vi "osciloscope.vi"() -> ()   [LabVIEW 2023]
doc: "Simulate a osciloscope VI"
uses:
  <vilib>/Utility/error.llb/DialogType.ctl
  <vilib>/Analysis/Matrix/Numeric/Conversions/Array To Matrix - RA.vi
  <vilib>/Analysis/Matrix/NI_Matrix.lvlib
panel:
  out "error out":errorcluster
  in  "error in (no error)":errorcluster
  in  "Stop":bool
  in  "Channel 2":bool
  in  "Y Position Channel-2":dbl(knob) scale=-5.0..5.0
  in  "X position":dbl(knob) step=1.0 scale=0.0..10.0
  in  "Mode":T1(ring)
  in  "Channel 1":bool
  in  "Y Position Channel-1":dbl(knob) scale=-5.0..5.0
  in  "Power":bool
  in  "Fetch":bool
  out "Scope":dbl[][](graph)
  # "Measurement"
  # "ON"
  # "OFF"
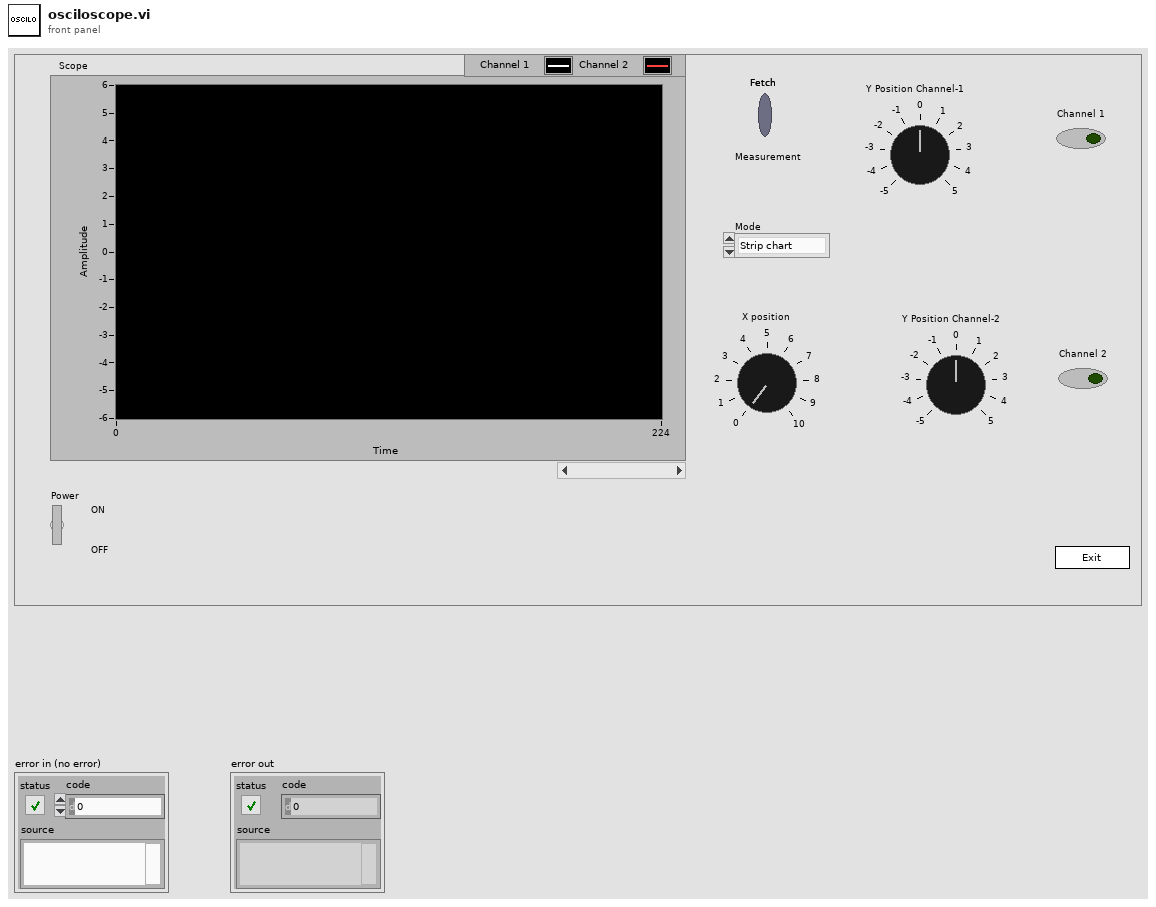
[diagram p1: front panel]
types:
  T1 = enum8{"Strip chart", "Scope chart", "Sweep chart"}
  T2 = cluster{"Power":bool, "Fetch":bool, "Channel 1":bool, "Channel 2":bool, "Y Channel 1":dbl, "Y Channel 2":dbl, "X Position":dbl, "x_value":i32}
  T3 = typedef "NI_Matrix.lvlib/RealMatrix.ctl" = dbl[][]
  T4 = typedef "DialogType.ctl" = u16
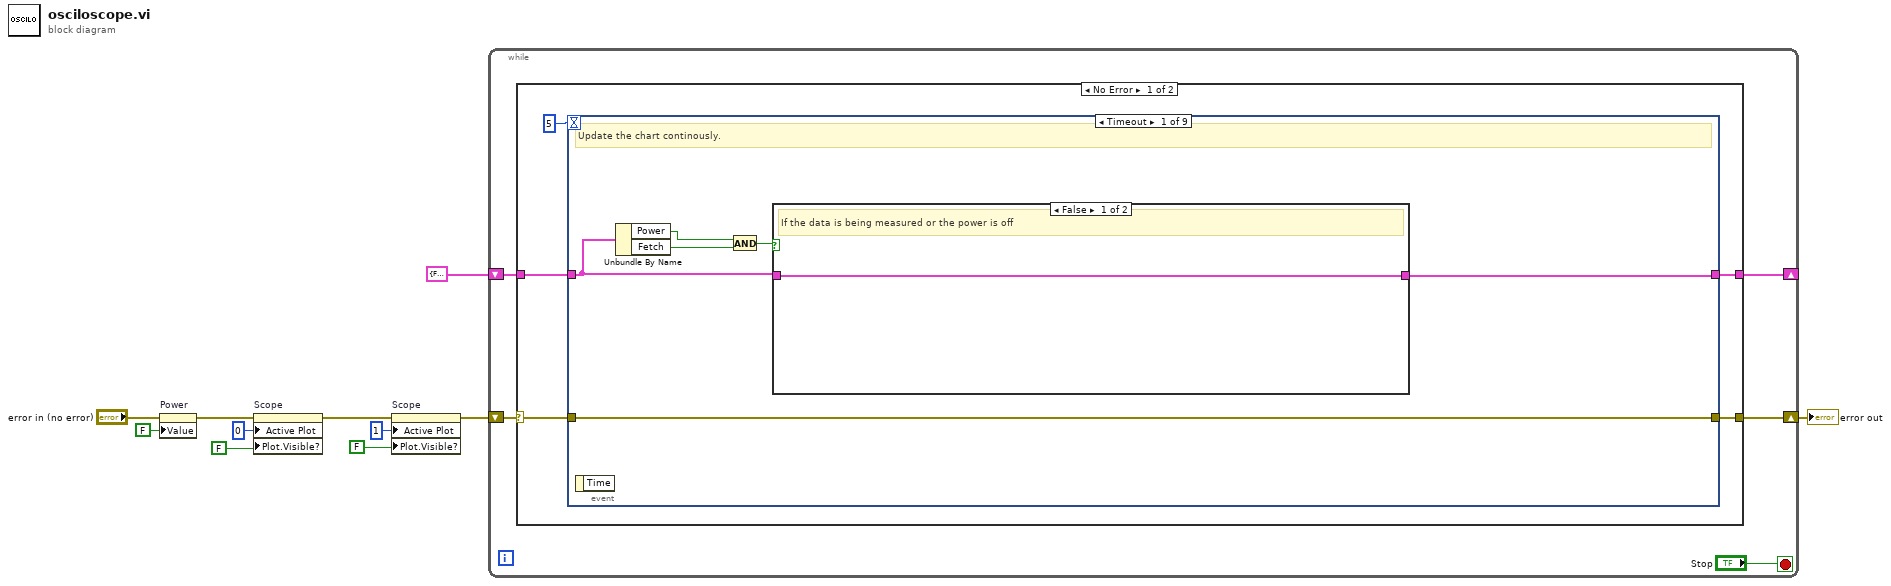
[diagram p0: block diagram]
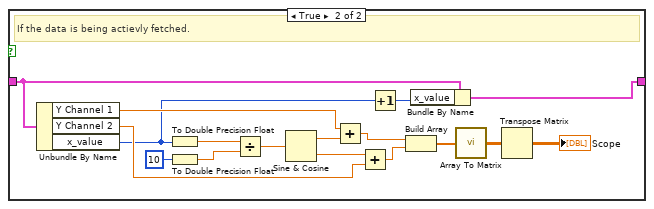
[diagram p2: hidden frame]
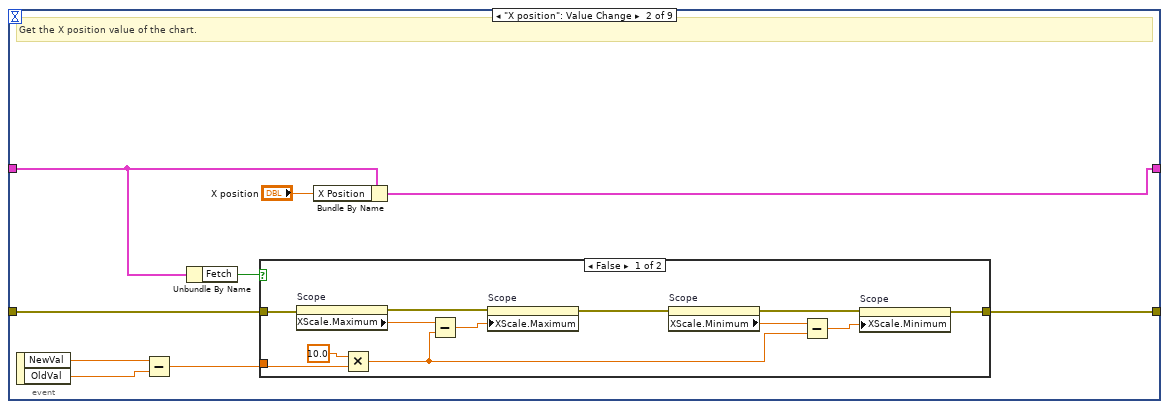
[diagram p3: hidden frame]
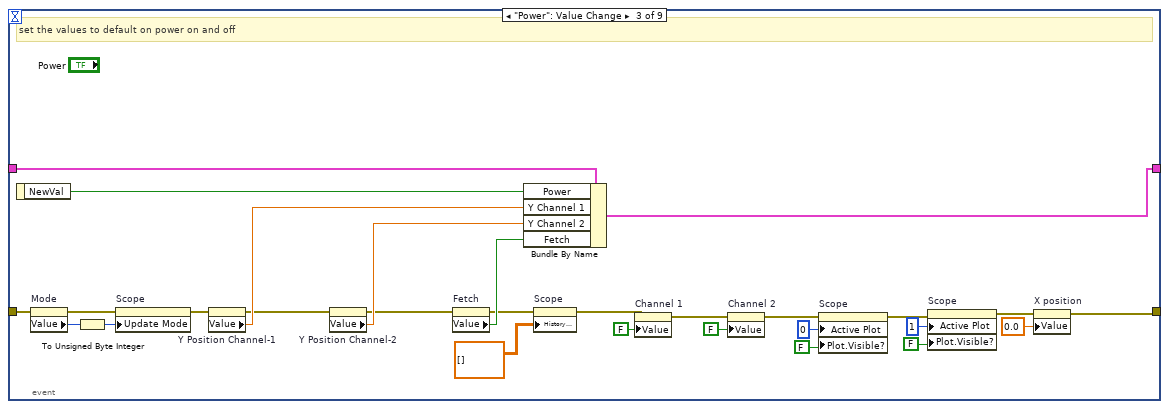
[diagram p5: hidden frame]
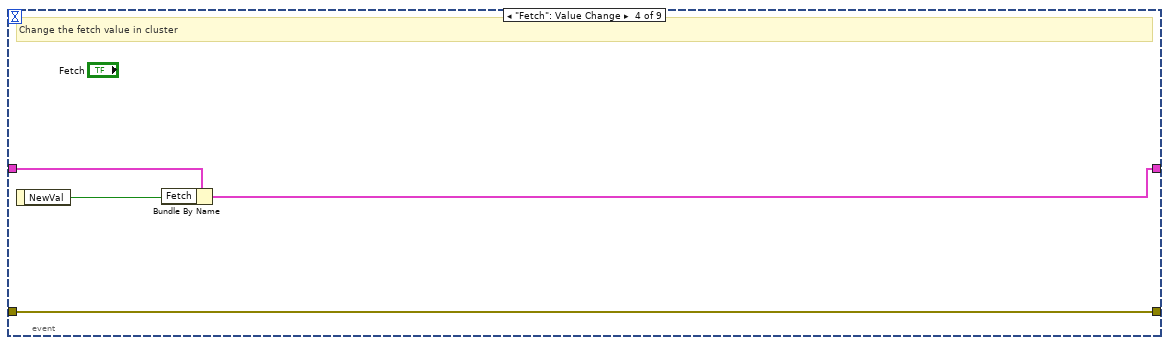
[diagram p6: hidden frame]
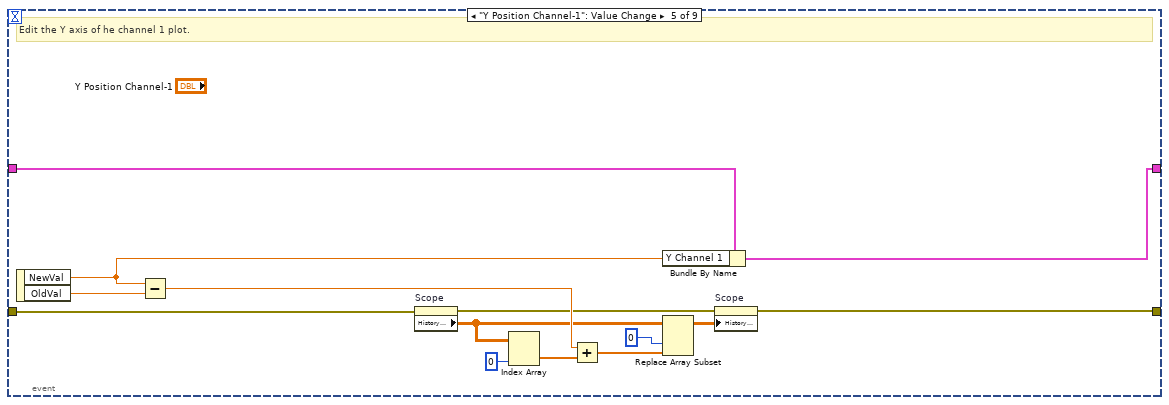
[diagram p7: hidden frame]
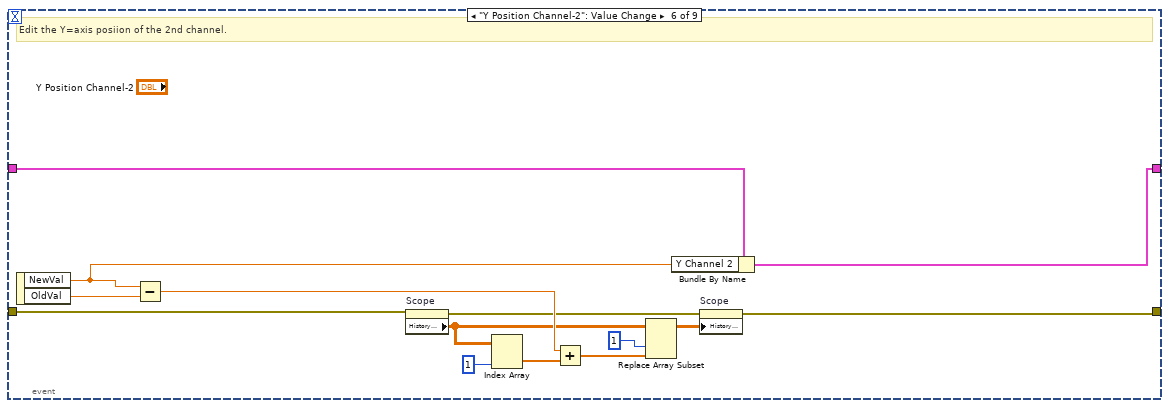
[diagram p8: hidden frame]
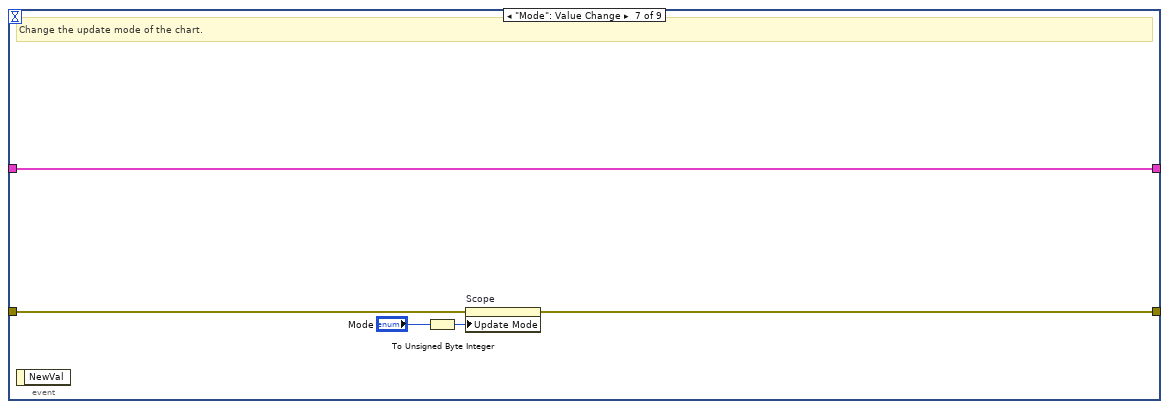
[diagram p9: hidden frame]
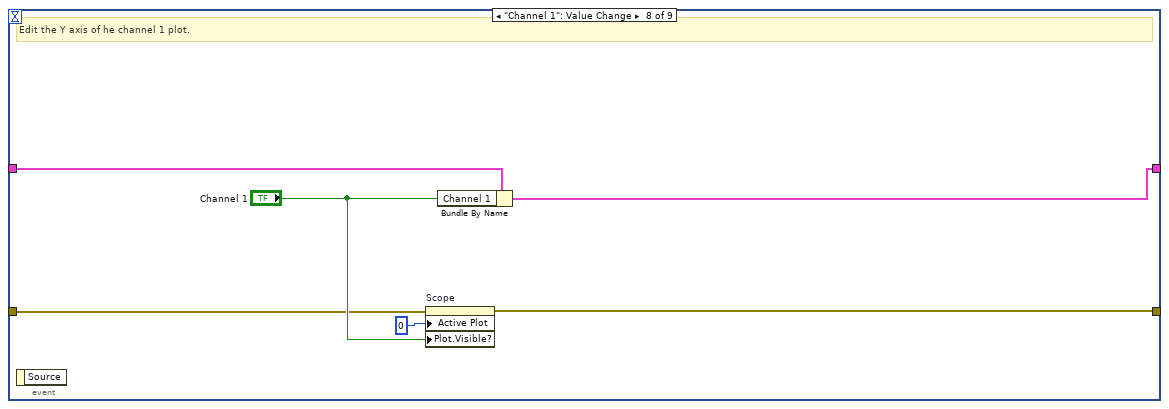
[diagram p10: hidden frame]
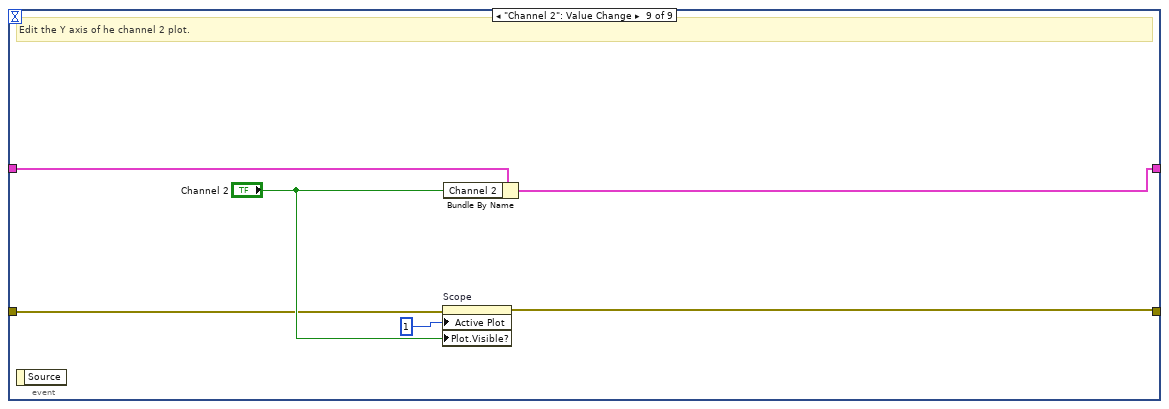
[diagram p11: hidden frame]
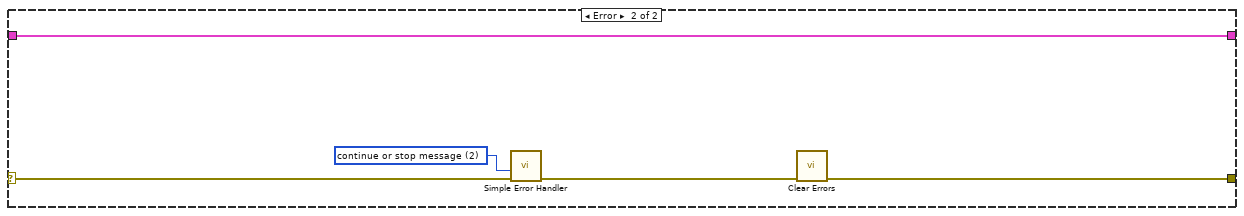
[diagram p12: hidden frame]
diagram:
  n1 = property on="Power" class="Bool (strict)"(error in="error in (no error)", "Value"=FALSE ("Power")) -> (error out=w4:errorcluster)  [unwired: 1 in, 1 out]
  n2 = property on="Scope" class="WFChart (strict)"(error in=w4, "Active Plot"=u32 0, "Plot.Visible?"=FALSE ("Plot.Visible")) -> (error out=w6:errorcluster)  [unwired: 1 in, 1 out]
  n3 = property on="Scope" class="WFChart (strict)"(error in=w6, "Active Plot"=u32 1, "Plot.Visible?"=FALSE ("Plot.Visible")) -> (error out=w3:errorcluster)  [unwired: 1 in, 1 out]
  n4 = while {
    shift-right: [w15] -> _
    shift-left: T2 {"Power"=FALSE, "Fetch"=TRUE, "Channel 1"=FALSE, "Channel 2"=FALSE, "Y Channel 1"=0.0, "Y Channel 2"=0.0, "X Position"=0.0, "x_value"=0} -> [w16]
    shift-right: [w12] -> w1
    shift-left: w3 -> [w13]
    stop <- "Stop" stop-if-true
    n5 = case shown="No Error" w13 {
      selector: w13 -> [w18 w148]
      tunnel: w16 -> [w20 w149]
      tunnel: [w19 w149] -> w15
      tunnel: [w17 w146] -> w12
      frame No Error {
        n6 = event shown="[0] Timeout" {
          selector: _ -> [_ _ _ _ _ _ _ _ _]
          dyn-events: _ -> [_ _ _ _ _ _ _ _ _]
          timeout: 5 ("milliseconds to wait") -> [_ _ _ _ _ _ _ _ _]
          tunnel: w20 -> [w27 w47 w95 w99 w110 w124 w131 w138 w144]
          tunnel: [w26 w54 w94 w98 w113 w127 w131 w137 w143] -> w19
          tunnel: w18 -> [w25 w50 w69 w96 w101 w115 w129 w134 w140]
          tunnel: [w25 w48 w68 w96 w100 w114 w128 w133 w139] -> w17
          event Timeout {
            # "Update the chart continously."
            n7 = event-data() -> ()  [unwired: 1 in, 1 out]
            n8 = Unbundle By Name(w27) -> ("Power"=w23:bool, "Fetch"=w22:bool)
            n9 = And(x=w23, y=w22) -> (x .and. y?=w24:bool)
            n10 = case shown="False" w24 {
              tunnel: w27 -> [w28 w32]
              tunnel: [w28 w31] -> w26
              frame False {
                # "If the data is being measured or the power is off"
              }
              frame True {
                # "If the data is being actievly fetched."
                n11 = Unbundle By Name(w32) -> ("Y Channel 1"=w34:dbl, "Y Channel 2"=w33:dbl, "x_value"=w29:i32)
                n12 = To Double Precision Float(number=w29) -> (double precision float=w43:dbl)
                n13 = To Double Precision Float(number=10 ("y")) -> (double precision float=w42:dbl)
                n14 = Divide(x=w43, y=w42) -> (x/y=w45:dbl)
                n15 = Sine & Cosine(0:w45) -> (1:w36:dbl, 2:w41:dbl)
                n16 = Add(x=w34, y=w36) -> (x+y=w37:dbl)
                n17 = Add(x=w41, y=w33) -> (x+y=w35:dbl)
                n18 = Increment(x=w29) -> (x+1=w30:i32)
                n19 = Build Array(w37, w35) -> (w39:dbl[])
                n20 = Bundle By Name(cluster=w32, "x_value"=w30) -> (w31:T2)
                n21 = call-poly <vilib>:"Array To Matrix.vi"("Real 1D Array"=w39) -> ("Real Matrix (Column Vector)"=w40:T3)
                n22 = Transpose Matrix(1:w40) -> (0:→"Scope":T3)
              }
            }
          }
          event "X position": Value Change {
            # "Get the X position value of the chart."
            n23 = event-data() -> ("NewVal"=w52:dbl, "OldVal"=w51:dbl)  [unwired: 1 in]
            n24 = Subtract(x=w52, y=w51) -> (x-y=w49:dbl)
            n25 = Unbundle By Name(w47) -> ("Fetch"=w46:bool)
            n26 = case shown="False" w46 {
              tunnel: w50 -> [w64 w67]
              tunnel: w49 -> [w62 _]
              tunnel: [w56 w67] -> w48
              frame False {
                n27 = property on="Scope" class="WFChart (strict)"(error in=w64) -> (error out=w63:errorcluster, "XScale.Maximum"=w65:dbl)  [unwired: 1 in, 1 out]
                n28 = Multiply(x=10.0, y=w62) -> (x*y=w55:dbl)
                n29 = Subtract(x=w65, y=w55) -> (x-y=w66:dbl)
                n30 = property on="Scope" class="WFChart (strict)"(error in=w63, "XScale.Maximum"=w66) -> (error out=w57:errorcluster)  [unwired: 1 in, 1 out]
                n31 = property on="Scope" class="WFChart (strict)"(error in=w57) -> (error out=w60:errorcluster, "XScale.Minimum"=w59:dbl)  [unwired: 1 in, 1 out]
                n32 = Subtract(x=w59, y=w55) -> (x-y=w58:dbl)
                n33 = property on="Scope" class="WFChart (strict)"(error in=w60, "XScale.Minimum"=w58) -> (error out=w56:errorcluster)  [unwired: 1 in, 1 out]
              }
              frame True {
              }
            }
            n34 = Bundle By Name(cluster=w47, "X Position"="X position") -> (w54:T2)
          }
          event "Power": Value Change {
            w70 = 0.0 items=["0", "1", "2", "3", "4", "5", "6", "7", "8", "9", "10"] ("X position")
            # "set the values to default on power on and off"
            n35 = event-data() -> ("NewVal"=w93:bool)  [unwired: 1 in]
            n36 = property on="Mode" class="Enum (strict)"(error in=w69) -> (error out=w88:errorcluster, "Value"=w89:T1)  [unwired: 1 in, 1 out]
            n37 = To Unsigned Byte Integer(number=w89) -> (unsigned 8bit integer=w90:u8)
            n38 = property on="Scope" class="WFChart (strict)"(error in=w88, "Update Mode"=w90) -> (error out=w83:errorcluster)  [unwired: 1 in, 1 out]
            n39 = property on="Y Position Channel-1" class="Knob (strict)"(error in=w83) -> (error out=w85:errorcluster, "Value"=w92:dbl)  [unwired: 1 in, 1 out]
            n40 = property on="Y Position Channel-2" class="Knob (strict)"(error in=w85) -> (error out=w86:errorcluster, "Value"=w91:dbl)  [unwired: 1 in, 1 out]
            n41 = property on="Fetch" class="Bool (strict)"(error in=w86) -> (error out=w84:errorcluster, "Value"=w87:bool)  [unwired: 1 in, 1 out]
            n42 = Bundle By Name(cluster=w95, "Power"=w93, "Y Channel 1"=w92, "Y Channel 2"=w91, "Fetch"=w87) -> (w94:T2)
            n43 = property on="Scope" class="WFChart (strict)"(error in=w84, "History Data"=dbl[][] []) -> (error out=w78:errorcluster)  [unwired: 1 in, 1 out]
            n44 = property on="Channel 1" class="Bool (strict)"(error in=w78, "Value"=FALSE ("Channel 1")) -> (error out=w81:errorcluster)  [unwired: 1 in, 1 out]
            n45 = property on="Channel 2" class="Bool (strict)"(error in=w81, "Value"=FALSE ("Channel 2")) -> (error out=w77:errorcluster)  [unwired: 1 in, 1 out]
            n46 = property on="Scope" class="WFChart (strict)"(error in=w77, "Active Plot"=u32 0, "Plot.Visible?"=FALSE ("Plot.Visible")) -> (error out=w76:errorcluster)  [unwired: 1 in, 1 out]
            n47 = property on="Scope" class="WFChart (strict)"(error in=w76, "Active Plot"=u32 1, "Plot.Visible?"=FALSE ("Plot.Visible")) -> (error out=w71:errorcluster)  [unwired: 1 in, 1 out]
            n48 = property on="X position" class="Knob (strict)"(error in=w71, "Value"=w70) -> (error out=w68:errorcluster)  [unwired: 1 in, 1 out]
          }
          event "Fetch": Value Change {
            # "Change the fetch value in cluster"
            n49 = event-data() -> ("NewVal"=w97:bool)  [unwired: 1 in]
            n50 = Bundle By Name(cluster=w99, "Fetch"=w97) -> (w98:T2)
          }
          event "Y Position Channel-1": Value Change {
            # "Edit the Y axis of he channel 1 plot."
            n51 = event-data() -> ("NewVal"=w109:dbl, "OldVal"=w111:dbl)  [unwired: 1 in]
            n52 = Subtract(x=w109, y=w111) -> (x-y=w112:dbl)
            n53 = property on="Scope" class="WFChart (strict)"(error in=w101) -> (error out=w103:errorcluster, "History Data"=w104:dbl[][])  [unwired: 1 in, 1 out]
            n54 = Index Array(array=w104, index (col)=0 ("disabled index (col)")) -> (element=w105:dbl[])  [unwired: 1 in]
            n55 = Add(x=w112, y=w105) -> (x+y=w106:dbl[])
            n56 = Bundle By Name(cluster=w110, "Y Channel 1"=w109) -> (w113:T2)
            n57 = Replace Array Subset(array=w104, new element=w106, index (col)=0 ("disabled index (col)")) -> (w102:dbl[][])  [unwired: 1 in]
            n58 = property on="Scope" class="WFChart (strict)"(error in=w103, "History Data"=w102) -> (error out=w100:errorcluster)  [unwired: 1 in, 1 out]
          }
          event "Y Position Channel-2": Value Change {
            # "Edit the Y=axis posiion of the 2nd channel."
            n59 = event-data() -> ("NewVal"=w116:dbl, "OldVal"=w125:dbl)  [unwired: 1 in]
            n60 = Subtract(x=w116, y=w125) -> (x-y=w126:dbl)
            n61 = property on="Scope" class="WFChart (strict)"(error in=w115) -> (error out=w117:errorcluster, "History Data"=w118:dbl[][])  [unwired: 1 in, 1 out]
            n62 = Index Array(array=w118, index (col)=1 ("disabled index (col)")) -> (element=w120:dbl[])  [unwired: 1 in]
            n63 = Add(x=w126, y=w120) -> (x+y=w121:dbl[])
            n64 = Replace Array Subset(array=w118, new element=w121, index (col)=1 ("disabled index (col)")) -> (w119:dbl[][])  [unwired: 1 in]
            n65 = Bundle By Name(cluster=w124, "Y Channel 2"=w116) -> (w127:T2)
            n66 = property on="Scope" class="WFChart (strict)"(error in=w117, "History Data"=w119) -> (error out=w114:errorcluster)  [unwired: 1 in, 1 out]
          }
          event "Mode": Value Change {
            # "Change the update mode of the chart."
            n67 = event-data() -> ()  [unwired: 1 in, 1 out]
            n68 = To Unsigned Byte Integer(number="Mode") -> (unsigned 8bit integer=w130:u8)
            n69 = property on="Scope" class="WFChart (strict)"(error in=w129, "Update Mode"=w130) -> (error out=w128:errorcluster)  [unwired: 1 in, 1 out]
          }
          event "Channel 1": Value Change {
            # "Edit the Y axis of he channel 1 plot."
            n70 = event-data() -> ()  [unwired: 1 in, 1 out]
            n71 = property on="Scope" class="WFChart (strict)"(error in=w134, "Active Plot"=u32 0, "Plot.Visible?"="Channel 1") -> (error out=w133:errorcluster)  [unwired: 1 in, 1 out]
            n72 = Bundle By Name(cluster=w138, "Channel 1"="Channel 1") -> (w137:T2)
          }
          event "Channel 2": Value Change {
            # "Edit the Y axis of he channel 2 plot."
            n73 = event-data() -> ()  [unwired: 1 in, 1 out]
            n74 = property on="Scope" class="WFChart (strict)"(error in=w140, "Active Plot"=u32 1, "Plot.Visible?"="Channel 2") -> (error out=w139:errorcluster)  [unwired: 1 in, 1 out]
            n75 = Bundle By Name(cluster=w144, "Channel 2"="Channel 2") -> (w143:T2)
          }
        }
      }
      frame Error {
        w145 = T4 2 items=["no dialog", "OK message", "continue or stop message", "OK message + warnings", "continue/stop + warnings"] ("type of dialog (OK msg:1)")
        n76 = call <vilib>:"Simple Error Handler.vi"("type of dialog (OK msg:1)"=w145, "error in (no error)"=w148) -> ("error out"=w147:errorcluster)  [unwired: 3 in, 4 out]
        n77 = call <vilib>:"Clear Errors.vi"("error in (no error)"=w147) -> ("error out"=w146:errorcluster)  [unwired: 5 in, 1 out]
      }
    }
  }
  "error out" <- w1
